vi "readLasers.vi"(7 "Reset Count":bool, 8 "Laser 2":bool, 9 "Laser 1":bool, 10 "Fancy Laser 2":bool, 11 "Fancy Laser 1":bool) -> (2 "Laser Readings":T1)   [LabVIEW 2014]
uses:
  Type Defs/laserReading.ctl
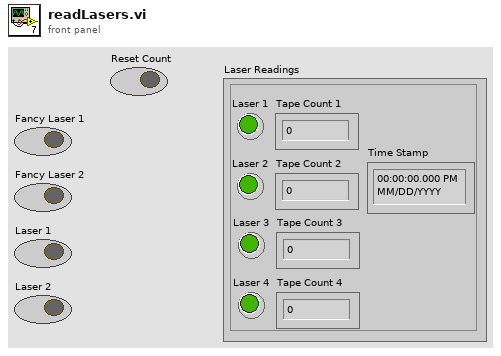
[diagram p1: front panel]
types:
  T1 = typedef "laserReading.ctl" = cluster{"Laser 1":bool, "Tape Count 1":u32, "Laser 2":bool, "Tape Count 2":u32, "Laser 3":bool, "Tape Count 3":u32, "Laser 4":bool, "Tape Count 4":u32, "Time Stamp":timestamp}
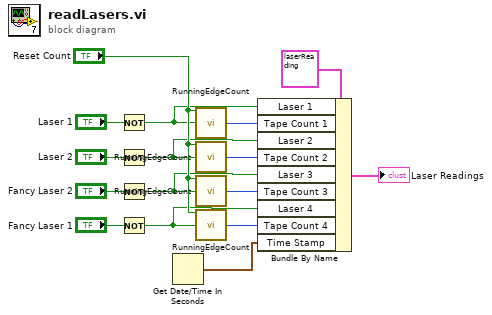
[diagram p0: block diagram]
diagram:
  n1 = Not(x="Laser 1") -> (.not. x?=w4:bool)
  n2 = Not(x="Laser 2") -> (.not. x?=w3:bool)
  n3 = Not(x="Fancy Laser 2") -> (.not. x?=w2:bool)
  n4 = Not(x="Fancy Laser 1") -> (.not. x?=w1:bool)
  n5 = Get Date/Time In Seconds() -> (seconds since 1Jan1904=w16:timestamp)
  n6 = call "RunningEdgeCount.vi"("Reset Count? (F)"="Reset Count", "Input"=w4) -> ("Count"=w9:u32)  [unwired: 3 in]
  n7 = call "RunningEdgeCount.vi"("Reset Count? (F)"="Reset Count", "Input"=w3) -> ("Count"=w7:u32)  [unwired: 3 in]
  n8 = call "RunningEdgeCount.vi"("Reset Count? (F)"="Reset Count", "Input"=w2) -> ("Count"=w6:u32)  [unwired: 3 in]
  n9 = call "RunningEdgeCount.vi"("Reset Count? (F)"="Reset Count", "Input"=w1) -> ("Count"=w8:u32)  [unwired: 3 in]
  n10 = Bundle By Name(cluster=T1 {"Laser 1"=FALSE, "Tape Count 1"=0, "Laser 2"=FALSE, "Tape Count 2"=0, "Laser 3"=FALSE, "Tape Count 3"=0, "Laser 4"=FALSE, "Tape Count 4"=0, "Time Stamp"=timestamp(0 s since 1904-01-01)} ("Laser Readings"), "Laser 1"=w4, "Tape Count 1"=w9, "Laser 2"=w3, "Tape Count 2"=w7, "Laser 3"=w2, "Tape Count 3"=w6, "Laser 4"=w1, "Tape Count 4"=w8, "Time Stamp"=w16) -> (→"Laser Readings":T1)
